vi "TrapProfile_Direct.vi"(9 "Direction":i32, 11 "in TRAPEZOID_PROFILE_STATE":T1 {"Velocity" format="%16_6e"; "Position" format="%16_6e"}) -> (3 "out TRAPEZOID_PROFILE_STATE":T1 {"Velocity" format="%16_6e"; "Position" format="%16_6e"})   [LabVIEW 2019, in "Trajectory_Library.lvlib"]
doc: "DO NOT USE. THIS IS AN INTERNAL ONLY ROUTINE.\n\nFlip the sign of the velocity and position if the profile is inverted\n\nInputs:\n - State -- Trapezoid Profile State\n - Direction -- SIgn value (-1, 1)\n\nOutputs:\n - State -- Updated Trapezoid Profile State"
uses:
  Trajectory_Library.lvlib
  TypeDef/TRAPEZOID_PROFILE_STATE.ctl
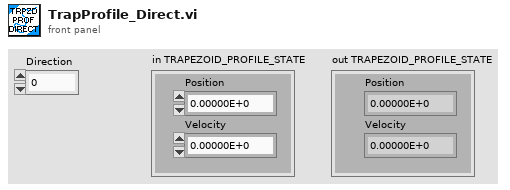
[diagram p1: front panel]
types:
  T1 = typedef "Trajectory_Library.lvlib/TRAPEZOID_PROFILE_STATE.ctl" = cluster{"Position":dbl, "Velocity":dbl}
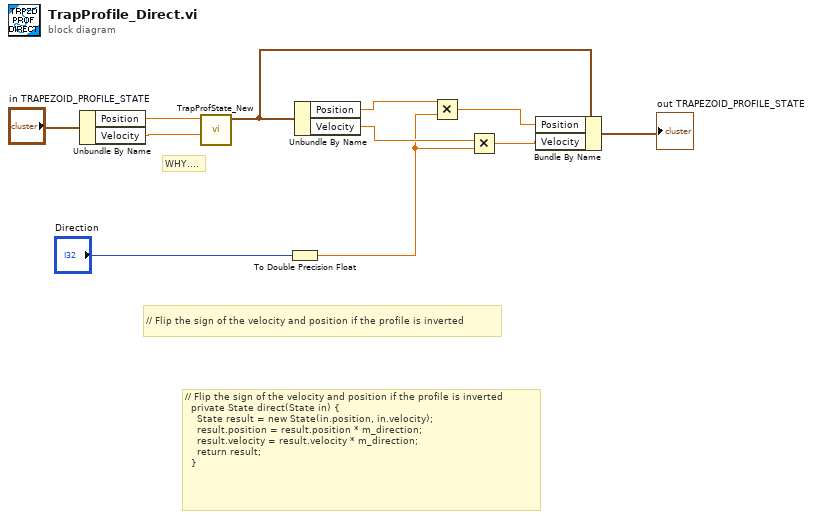
[diagram p0: block diagram]
diagram:
  # "// Flip the sign of the velocity and position if the profile is inverted\n  private State direct(State in) {\n    State result = new State(in.position, in.velocity);\n    result.position = result.position * m_direction;\n    result.velocity = result.velocity * m_direction;\n    return result;\n  }"
  # "WHY...."
  # "// Flip the sign of the velocity and position if the profile is inverted"
  n1 = Unbundle By Name("in TRAPEZOID_PROFILE_STATE") -> ("Position"=w10:dbl, "Velocity"=w9:dbl)
  n2 = call "TrapProfState_New.vi"("Velocity"=w9, "Position"=w10) -> ("TRAPEZOID_PROFILE_STATE"=w8:T1)  [unwired: 9 in]
  n3 = To Double Precision Float(number="Direction") -> (double precision float=w2:dbl)
  n4 = Unbundle By Name(w8) -> ("Position"=w5:dbl, "Velocity"=w4:dbl)
  n5 = Multiply(x=w5, y=w2) -> (x*y=w6:dbl)
  n6 = Multiply(x=w4, y=w2) -> (x*y=w7:dbl)
  n7 = Bundle By Name(cluster=w8, "Position"=w6, "Velocity"=w7) -> (→"out TRAPEZOID_PROFILE_STATE":T1)
